vi "Trav-Stop.vi"(10 "Settings":T2) -> ()   [LabVIEW 2017]
uses:
  TypeDefs/Trav-Command-TD.ctl
  TypeDefs/Position-Info-TD.ctl
  Settings/Settings-Control.ctl
panel:
  in  "Position Info IN":T1
  out "Position Info OUT":T1
  in  "Trav Command":T3 items=["Set Reference", "Read Position", "Move", "StopMotors"]
  out "error out":errorcluster
  in  "error in":errorcluster
  in  "Stop Button":bool
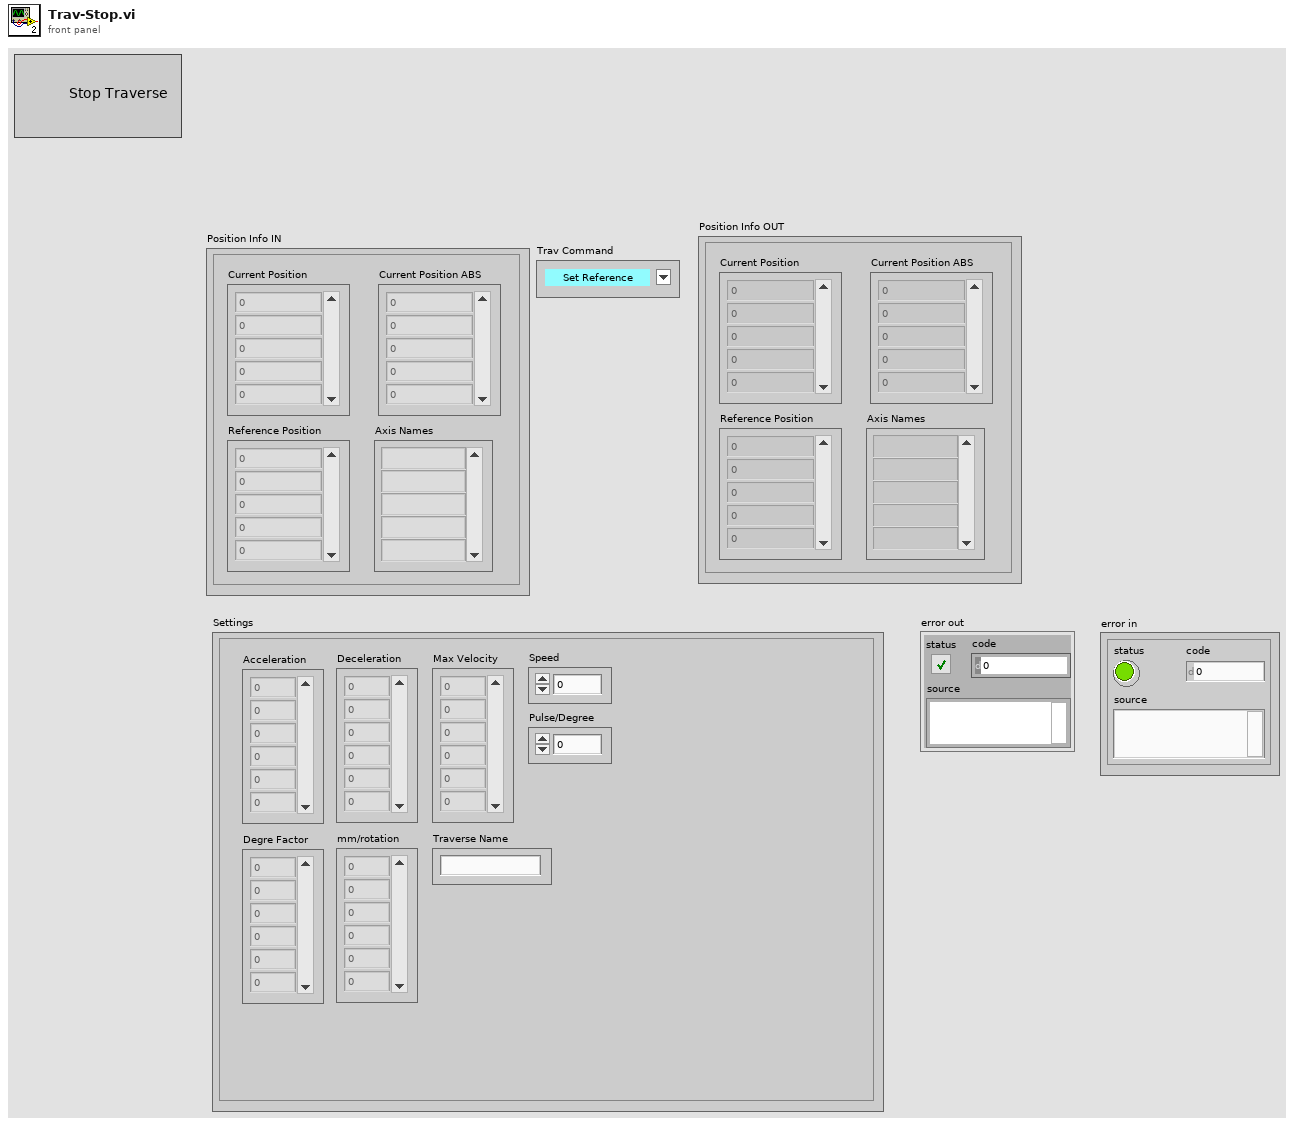
[diagram p1: front panel]
types:
  T1 = typedef "Position-Info-TD.ctl" = cluster{"Current Position ABS":dbl[], "Current Position":dbl[], "Reference Position":dbl[], "Axis Names":string[]}
  T2 = typedef "Settings-Control.ctl" = cluster{"Acceleration":dbl[], "Deceleration":dbl[], "Max Velocity":dbl[], "Speed":dbl, "Pulse/Degree":dbl, "Degre Factor":dbl[], "mm/rotation":dbl[], "Traverse Name":string}
  T3 = typedef "Trav-Command-TD.ctl" = u16
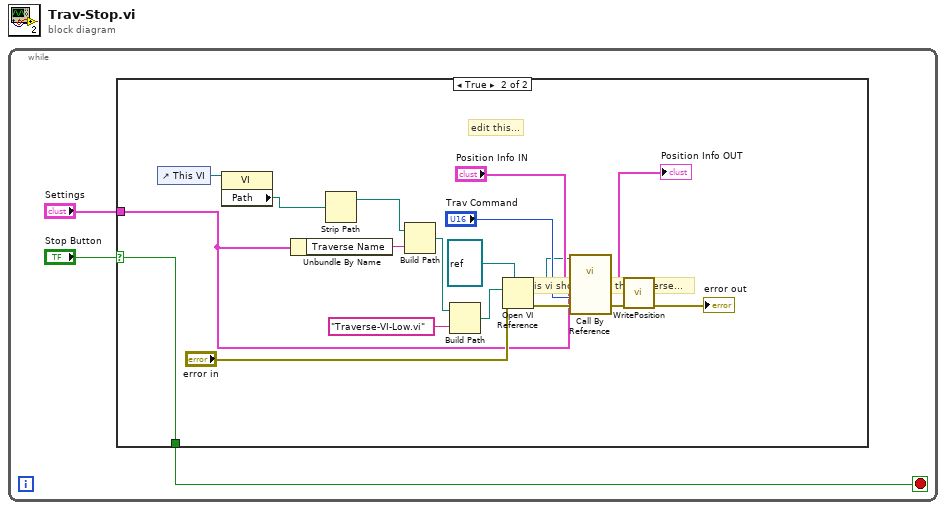
[diagram p0: block diagram]
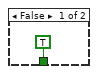
[diagram p2: hidden frame]
diagram:
  n1 = while {
    stop <- w2 stop-if-true
    n2 = case shown="True" "Stop Button" {
      selector: "Stop Button" -> [_ w6]
      tunnel: [TRUE w6] -> w2
      tunnel: "Settings" -> [_ w5]
      frame False {
      }
      frame True {
        # "this vi should stop the traverse..."
        # "edit this..."
        n3 = control-ref of="This VI"() -> (w15:refnum<vi>)
        n4 = property class="VI"(reference=w15) -> ("Path"=w14:path)  [unwired: 1 in, 2 out]
        n5 = Unbundle By Name(w5) -> ("Traverse Name"=w17:string)
        n6 = Strip Path(path=w14) -> (stripped path=w16:path)  [unwired: 1 out]
        n7 = Build Path(base path=w16, name or relative path=w17) -> (appended path=w18:path)
        n8 = Build Path(base path=w18, name or relative path="Traverse-VI-Low.vi") -> (appended path=w20:path)
        n9 = Open VI Reference(type specifier VI Refnum (for type only)=refnum<vi> refnum, vi path=w20, error in (no error)="error in") -> (vi reference=w8:refnum<vi>, error out=w11:errorcluster)  [unwired: 3 in]
        n10 = call-by-ref "?"(reference=w8, "error in"=w11, "Trav Command"="Trav Command", "Settings"=w5, "Position Info IN"="Position Info IN") -> ("error out"=w12:errorcluster, "Position Info OUT"=w10:T1)  [unwired: 7 in, 2 out]
        "Position Info OUT" <- w10
        n11 = call "WritePosition.vi"("error in"=w12, "Position Info"=w10) -> ("error out"=→"error out":errorcluster)  [unwired: 9 in]
      }
    }
  }
